vi "picoscopeParseTraceData.vi"(6 "Sample Rate":sgl, 9 "MultiBuffers (Max or non-aggregated)":T2(array[cluster]), 10 "Display Buffer Index":i32, 11 "PicoscopeV2 in":refnum<class "PicoscopeV2.lvclass">) -> (2 "Array":cluster{i32, sgl, "Data":dbl[]}[](array[cluster]), 3 "PicoscopeV2 out":refnum<class "PicoscopeV2.lvclass">)   [LabVIEW 2020, in "PicoscopeV2.lvclass"]
uses:
  PicoscopeV2.lvclass
  PicoscopeV2.lvclass/PicoscopeV2.ctl
panel:
  out "GEECS waveforms info":T1(array[cluster])
  out "scope traces":i16[][](array[numeric])
  out "appended array":waveform(dbl)[](array[waveform])
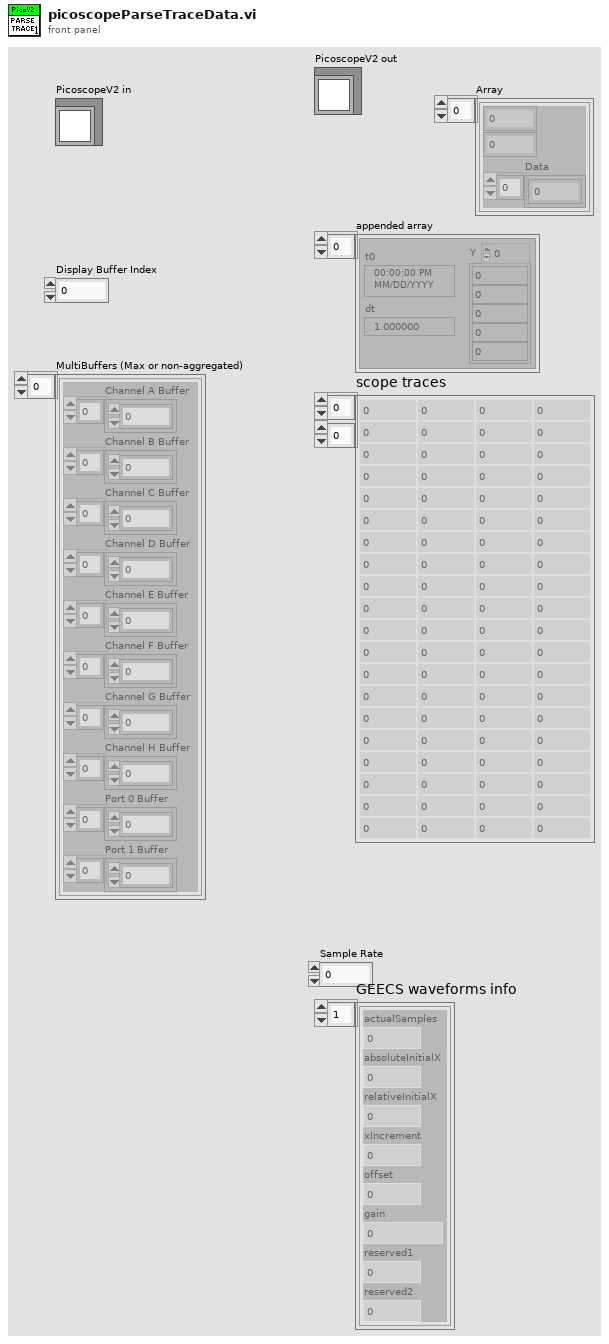
[diagram p1: front panel]
types:
  T1 = cluster{"actualSamples":i32, "absoluteInitialX":dbl, "relativeInitialX":dbl, "xIncrement":dbl, "offset":dbl, "gain":dbl, "reserved1":dbl, "reserved2":dbl}[]
  T2 = cluster{"Channel A Buffer":i16[], "Channel B Buffer":i16[], "Channel C Buffer":i16[], "Channel D Buffer":i16[], "Channel E Buffer":i16[], "Channel F Buffer":i16[], "Channel G Buffer":i16[], "Channel H Buffer":i16[], "Port 0 Buffer":i16[], "Port 1 Buffer":i16[]}[]
  T3 = cluster{"Channel0":string, "Channel1":string, "Channel2":string, "Channel3":string, "Channel4":string, "Channel5":string, "Channel6":string, "Channel7":string}
  T4 = cluster{"NumberofChannels":dbl, "GUInumPoints":i32}
  T5 = typedef "PicoScope5000aAnalogChannelSettings.ctl" = cluster{"Enabled":bool, "Coupling":i16, "Range":u16, "Analogue Offset":sgl, "Bandwidth Limit":u32}
  T6 = cluster{"Channel A Buffer":i16[], "Channel B Buffer":i16[], "Channel C Buffer":i16[], "Channel D Buffer":i16[], "Channel E Buffer":i16[], "Channel F Buffer":i16[], "Channel G Buffer":i16[], "Channel H Buffer":i16[], "Port 0 Buffer":i16[], "Port 1 Buffer":i16[]}
  T7 = typedef "OnOffTypeDef.ctl" = enum16{"off", "on"}
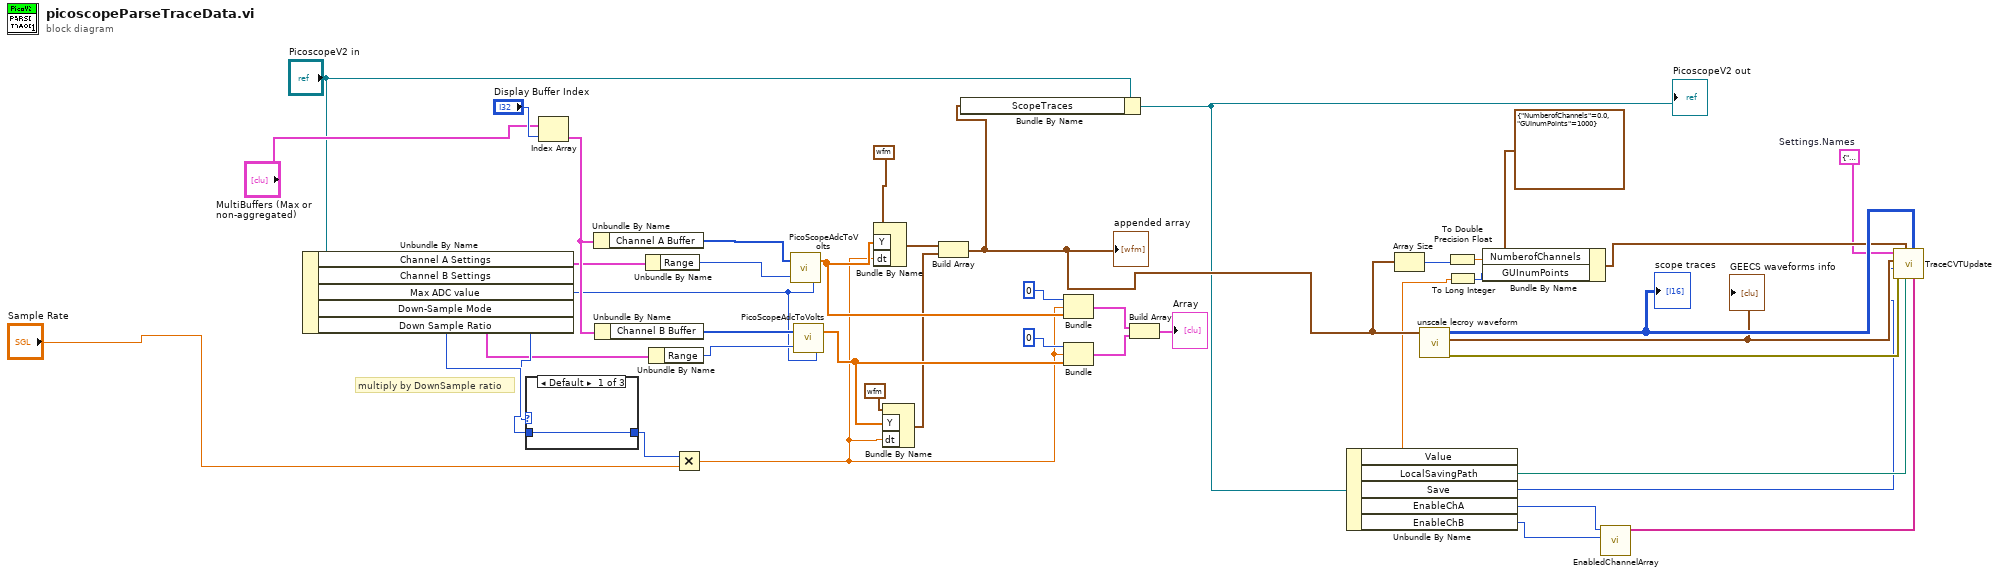
[diagram p0: block diagram]
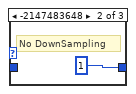
[diagram p2: hidden frame]
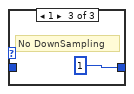
[diagram p3: hidden frame]
diagram:
  w5 = T3 {"Channel0"="Channel0", "Channel1"="Channel1", "Channel2"="Channel2", "Channel3"="Channel3", "Channel4"="", "Channel5"="", "Channel6"="", "Channel7"=""}  # Settings.Names
  # "multiply by DownSample ratio"
  n1 = Unbundle By Name("PicoscopeV2 in") -> ("Channel A Settings"=w29:T5, "Channel B Settings"=w30:T5, "Max ADC value"=w31:i16, "Down-Sample Mode"=w43:u32, "Down Sample Ratio"=w44:u64)
  n2 = case shown="Default" w43 {
    tunnel: [w45 u64 1 ("Down Sample Ratio") u64 1 ("Down Sample Ratio")] -> w26
    tunnel: w44 -> [w45 _ _]
    frame Default {
    }
    frame -2147483648 {
      # "No DownSampling"
    }
    frame 1 {
      # "No DownSampling"
    }
  }
  n3 = Index Array(array="MultiBuffers (Max or non-aggregated)", index="Display Buffer Index") -> (element=w41:T6)
  n4 = Unbundle By Name(w41) -> ("Channel A Buffer"=w39:i16[])
  n5 = Unbundle By Name(w41) -> ("Channel B Buffer"=w35:i16[])
  n6 = Unbundle By Name(w29) -> ("Range"=w33:u16)
  n7 = Unbundle By Name(w30) -> ("Range"=w42:u16)
  n8 = Multiply(x=w26, y="Sample Rate") -> (x*y=w21:sgl)
  n9 = call "PicoScopeAdcToVolts.vi"("Max_adc"=w31, "Range Index"=w33, "Data"=w39) -> ("Data"=w22:dbl[])
  n10 = call "PicoScopeAdcToVolts.vi"("Max_adc"=w31, "Range Index"=w42, "Data"=w35) -> ("Data"=w25:dbl[])
  n11 = Bundle By Name(cluster=waveform(dbl) {"t0"=timestamp(0 s since 1904-01-01), "dt"=1.0, "Y"=[]} ("waveform"), "Y"=w22, "dt"=w21) -> (w20:waveform(dbl))
  n12 = Bundle By Name(cluster=waveform(dbl) {"t0"=timestamp(0 s since 1904-01-01), "dt"=1.0, "Y"=[]} ("waveform"), "Y"=w25, "dt"=w21) -> (w19:waveform(dbl))
  n13 = Build Array(w20, w19) -> (w17:waveform(dbl)[])
  "appended array" <- w17
  n14 = Bundle By Name(cluster="PicoscopeV2 in", "ScopeTraces"=w17) -> (w16:refnum<class "PicoscopeV2.lvclass">)
  "PicoscopeV2 out" <- w16
  n15 = Bundle(0, w21, "Data"=w22) -> (w36:cluster{i32, sgl, "Data":dbl[]})  [unwired: 1 in]
  n16 = Bundle(0, w21, "Data"=w25) -> (w37:cluster{i32, sgl, "Data":dbl[]})  [unwired: 1 in]
  n17 = Build Array(w36, w37) -> (→"Array":cluster{i32, sgl, "Data":dbl[]}[])
  n18 = Unbundle By Name(w16) -> ("Value"=w13:dbl, "LocalSavingPath"=w6:path, "Save"=w4:T7, "EnableChA"=w3:T7, "EnableChB"=w2:T7)
  n19 = Array Size(array=w17) -> (size(s)=w11:i32)
  n20 = call "unscale lecroy waveform.vi"("Waveforms"=w17) -> ("Error out"=w7:errorcluster, "GEECS waveforms info"=w8:T1, "scope traces"=w10:i16[][])  [unwired: 8 in]
  "scope traces" <- w10
  "GEECS waveforms info" <- w8
  n21 = To Double Precision Float(number=w11) -> (double precision float=w12:dbl)
  n22 = To Long Integer(number=w13) -> (32bit integer=w14:i32)
  n23 = Bundle By Name(cluster=T4 {"NumberofChannels"=0.0, "GUInumPoints"=1000}, "NumberofChannels"=w12, "GUInumPoints"=w14) -> (w9:T4)
  n24 = call "EnabledChannelArray.vi"("Channel1"=w2, "Channel0"=w3) -> ("EnabledChannels"=w1:string[])  [unwired: 9 in]
  n25 = call "TraceCVTUpdate.vi"("Channels"=w1, "wfm"=w10, "Settings.LocalSavingPath"=w6, "TraceGUI-Info"=w9, "error in (no error)"=w7, "Save"=w4, "wfm info"=w8, "Settings.Names"=w5) -> ()  [unwired: 1 in, 3 out]
